vi "Global 1.vi"() -> ()   [LabVIEW 2016]
panel:
  out "camera?":bool
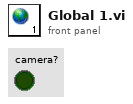
[diagram p1: front panel]
diagram:
